vi "Extract Image Center.vi"(8 "Zone Size":dbl=7.0 format="%#_13g", 9 "Exam Zone Offset Y":dbl, 10 "Exam Zone Offset X":dbl, 11 "Source In":T1) -> (2 "Extracted Out":T1, 3 "Annotated Source Out":T1)   [LabVIEW 2014]
uses:
  <vilib>/vision/Image Controls.llb/IMAQ Image.ctl
  <vilib>/vision/NI_Vision_Development_Module.lvlib
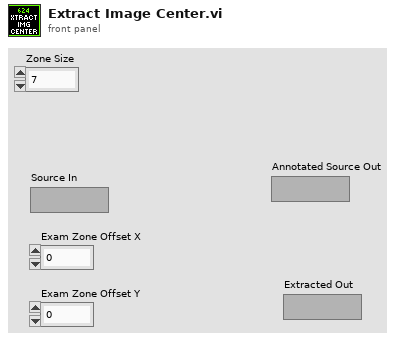
[diagram p1: front panel]
types:
  T1 = typedef "IMAQ Image.ctl" = refnum<image>
  T2 = typedef "Image Type" = u32
  T3 = cluster{"[0]":i32, "[1]":i32, "[2]":i32, "[3]":i32}
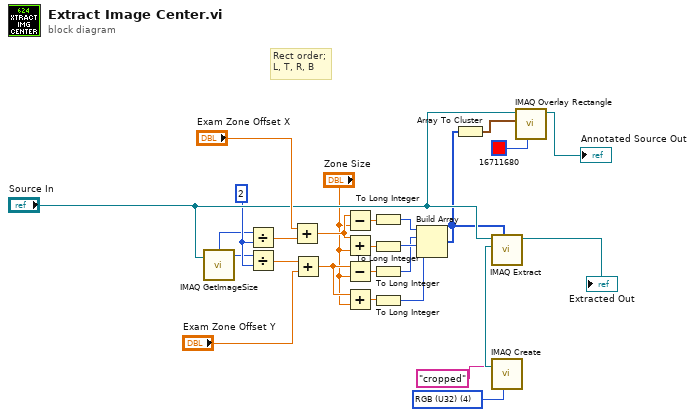
[diagram p0: block diagram]
diagram:
  w13 = T2 4 items=["Grayscale (U8)", "Grayscale (I16)", "Grayscale (SGL)", "Complex (CSG)", "RGB (U32)", "HSL (U32)", "RGB (U64)", "Grayscale (U16)"] ("Image Type")
  w3 = 2 ("y")
  # "Rect order;\nL, T, R, B"
  n1 = call "IMAQ GetImageSize"("Image"="Source In") -> ("Y Resolution"=w2:i32, "X Resolution"=w1:i32)  [unwired: 3 in, 1 out]
  n2 = Divide(x=w1, y=w3) -> (x/y=w21:dbl)
  n3 = Divide(x=w2, y=w3) -> (x/y=w23:dbl)
  n4 = Add(x="Exam Zone Offset X", y=w21) -> (x+y=w26:dbl)
  n5 = Add(x=w23, y="Exam Zone Offset Y") -> (x+y=w25:dbl)
  n6 = Subtract(x=w26, y="Zone Size") -> (x-y=w5:dbl)
  n7 = Add(x=w26, y="Zone Size") -> (x+y=w15:dbl)
  n8 = Subtract(x=w25, y="Zone Size") -> (x-y=w6:dbl)
  n9 = Add(x=w25, y="Zone Size") -> (x+y=w7:dbl)
  n10 = To Long Integer(number=w5) -> (32bit integer=w8:i32)
  n11 = To Long Integer(number=w15) -> (32bit integer=w10:i32)
  n12 = To Long Integer(number=w6) -> (32bit integer=w9:i32)
  n13 = To Long Integer(number=w7) -> (32bit integer=w11:i32)
  n14 = Build Array(w8, w9, w10, w11) -> (w16:i32[])
  n15 = Array To Cluster(array=w16) -> (cluster=w17:T3)
  n16 = call "IMAQ Create"("Image Name"="cropped", "Image Type"=w13) -> ("New Image"=w14:T1)  [unwired: 3 in, 1 out]
  n17 = call "IMAQ Extract"("Optional Rectangle"=w16, "Image Dst"=w14, "Image Src"="Source In") -> ("Image Dst Out"=→"Extracted Out":T1)  [unwired: 7 in, 1 out]
  n18 = call "IMAQ Overlay Rectangle"("Color"=u32 16711680, "Rectangle"=w17, "Image"="Source In") -> ("Image Out"=→"Annotated Source Out":T1)  [unwired: 7 in, 1 out]
